vi "Lock-in query OVLD.vi"(8 "error in (no error)":errorcluster, 11 "Lockin SR830.lvclass In":refnum<class "Lockin SR830.lvclass">) -> (0 "error out":errorcluster, 2 "Sensitivity":T1 items=["2 nV", "5 nV", "10 nV", "20 nV", "50 nV", "100 nV", "200 nV", "500 nV", "1 uV", "2 uV", "5 uV", "10 uV", "20 uV", "50 uV", "100 uV", "200 uV", "500 uV", "1 mV", "2 mV", "5 mV", "10 mV", "20 mV", "50 mV", "100 mV", "200 mV", "500 mV", "1 V"], 3 "Lockin SR830.lvclass out":refnum<class "Lockin SR830.lvclass">)   [LabVIEW 2017]
uses:
  Lockin SR830.lvclass
  Sensitivity.ctl
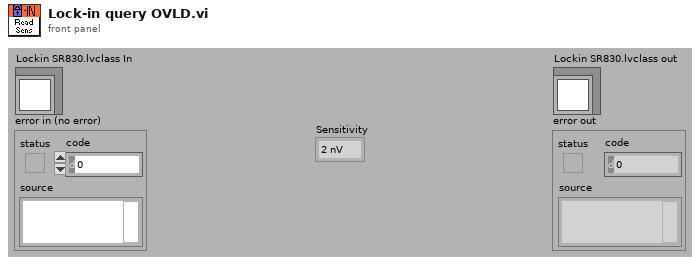
[diagram p1: front panel]
types:
  T1 = typedef "Lockin SR830.lvclass/Sensitivity.ctl" = u16
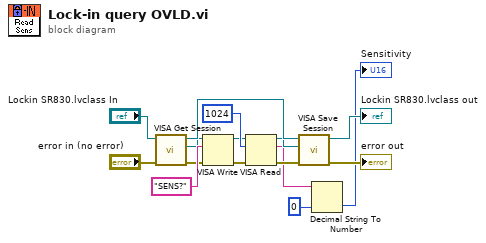
[diagram p0: block diagram]
diagram:
  n1 = call-dynamic "VISA Get Session.vi"("error in (no error)"="error in (no error)", "Instrument.lvclass in"="Lockin SR830.lvclass In") -> ("error out"=w7:errorcluster, "VISA Resource Name"=w8:refnum<visa-resource-name>, "Instrument.lvclass out"=w14:refnum<class "Lockin SR830.lvclass">)  [unwired: 6 in, 1 out]
  n2 = VISA Write(VISA resource name=w8, write buffer="SENS?" ("data"), error in (no error)=w7) -> (VISA resource name out=w4:refnum<visa-resource-name>, error out=w5:errorcluster)  [unwired: 1 out]
  n3 = VISA Read(VISA resource name=w4, byte count=u32 1024, error in (no error)=w5) -> (VISA resource name out=w3:refnum<visa-resource-name>, read buffer=w1:string, error out=w2:errorcluster)  [unwired: 1 out]
  n4 = call-dynamic "VISA Save Session.vi"("error in (no error)"=w2, "VISA Resource Name"=w3, "Instrument.lvclass in"=w14) -> ("error out"=→"error out":errorcluster, "Instrument.lvclass out"=→"Lockin SR830.lvclass out":refnum<class "Lockin SR830.lvclass">)  [unwired: 7 in]
  n5 = Decimal String To Number(string=w1, default (0L)=u16 0 ("default (0 I32)")) -> (number=→"Sensitivity":u16)  [unwired: 1 in, 1 out]
